vi "Check Sudoku Int by Formal.vi"(8 "error in (no error)":errorcluster, 11 "Sudoku Class in":refnum<class "Sudoku Class.lvclass">) -> (0 "error out":errorcluster, 1 "Is Modify":bool, 2 "Sudoku Int Out":u8[][](array[numeric]), 3 "Sudoku Class out":refnum<class "Sudoku Class.lvclass">)   [LabVIEW 2015, in "Sudoku Library.lvlib" / "Sudoku Class.lvclass"]
doc: "Created IvanLis by LabVIEW Portal\nProfile: http://labviewportal.org/memberlist.php?mode=viewprofile&u=987\neMail: IvanLisanov@gMail.com\nTelegram: https://t.me/IvanLis"
uses:
  Sudoku Class.lvclass
  Sudoku Class.lvclass/Sudoku Class.ctl
  Sudoku Library.lvlib
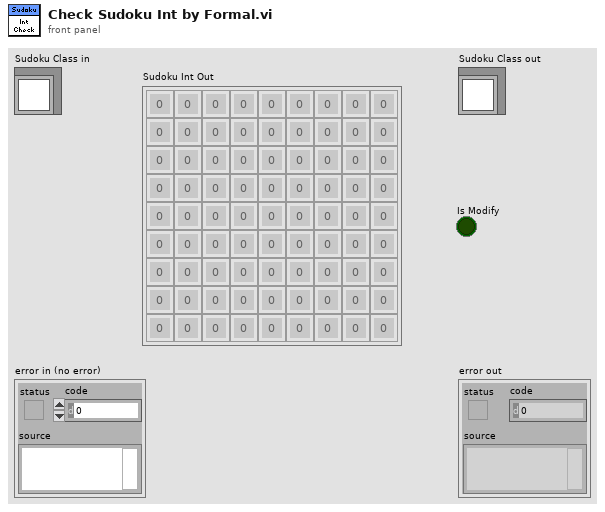
[diagram p1: front panel]
types:
  T1 = typedef "Sudoku Library.lvlib/Sudoku Formal.ctl" = T2[][]
  T2 = typedef "Sudoku Library.lvlib/Cell Formal.ctl" = cluster{"Variant":u8[]}
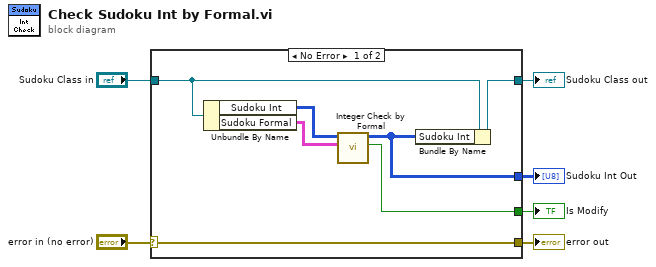
[diagram p0: block diagram]
diagram:
  n1 = case shown="No Error" "error in (no error)" {
    selector: "error in (no error)" -> [w13 w15]
    tunnel: [w13 w15] -> w5
    tunnel: [w11 w14] -> w3
    tunnel: "Sudoku Class in" -> [w12 w14]
    tunnel: [w7 _] -> w2
    tunnel: [w8 _] -> w1
    frame No Error {
      n2 = Unbundle By Name(w12) -> ("Sudoku Int"=w10:u8[][], "Sudoku Formal"=w9:T1)
      n3 = call "Integer Check by Formal.vi"("Sudoku Formal In"=w9, "Sudoku Int In"=w10) -> ("Is Modify"=w7:bool, "Sudoku Int Out"=w8:u8[][])  [unwired: 8 in]
      n4 = Bundle By Name(cluster=w12, "Sudoku Int"=w8) -> (w11:refnum<class "Sudoku Class.lvclass">)
    }
    frame Error {
    }
  }
  "error out" <- w5
  "Sudoku Class out" <- w3
  "Is Modify" <- w2
  "Sudoku Int Out" <- w1
